vi "Global.vi"() -> ()   [LabVIEW 2017]
uses:
  Control/Motor Position.ctl
  Control/Torque Vector.ctl
  Control/Virtual Damping.ctl
panel:
  out "Fitness Value":dbl
  in  "Virtual Damping":T1
  out "Leading":bool
  in  "MJT":cluster{"roll":dbl, "pitch":dbl, "yaw":dbl}={"roll"=-0.0, "pitch"=0.0, "yaw"=-0.0}
  in  "Torque Vector":T2
  in  "WayPoint":cluster{"roll":dbl, "pitch":dbl, "yaw":dbl}={"roll"=-0.0, "pitch"=0.0, "yaw"=-0.0}
  in  "EndEffector":cluster{"roll":dbl, "pitch":dbl, "yaw":dbl}
  out "Playback":bool
  in  "Stop":bool=TRUE
  in  "Motor Position":T3
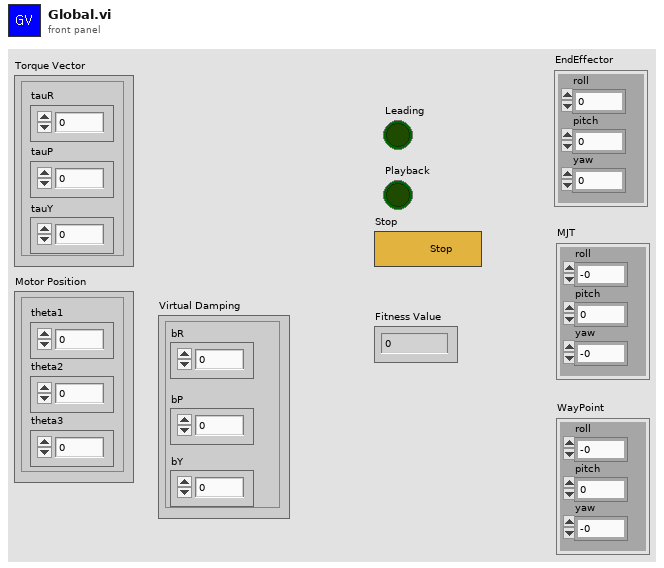
[diagram p1: front panel]
types:
  T1 = typedef "Virtual Damping.ctl" = cluster{"bR":dbl, "bP":dbl, "bY":dbl}
  T2 = typedef "Torque Vector.ctl" = cluster{"tauR":dbl, "tauP":dbl, "tauY":dbl}
  T3 = typedef "Motor Position.ctl" = cluster{"theta1":dbl, "theta2":dbl, "theta3":dbl}
diagram:
